vi "Teststand Post Sub Steps Read_FA_FE_FF_Frame STP_Engine.vi"(9 "Socket No":u16=1, 10 "STP Data in":T1={"ECU CAN Port"="CAN1", "CMD"=130, "CAN Write Data"=[], "Frame"="FE_FRAME_LOG", "Log"=TRUE} {"CMD" items=["TSW_VERSION(130)"=130, "WAIT_EVENT(132)"=132, "SEQUENCER(133)"=133, "TSW_RESET(150)"=150, "CONFIG_ECU(151)"=151, "TEST_CORE (152)"=152, "TEST_WATCHDOG (153)"=153, "TEST_MONITORING (154)"=154, "READ_MEMORY (162)"=162, "WRITE_ERASE_MEMORY (164)"=164, "COMM_EXTERNAL (190)"=190, "COMM_INTERNAL (195)"=195, "GET_ANALOG_INPUT (210)"=210, "GET_DIGITAL_INPUT (211)"=211, "GET_FREQUENCY_INPUT (212)"=212, "TEST_INPUT_STRUCTURE (214)"=214, "GENERATE_OUTPUT_SIGNAL (220)"=220, "GENERATE_SYNCHRONIZED_OUTPUT_SIGNALS (221)"=221, "eDCU_Specific (250)"=250]; "CAN Write Data" format="%.0x"}, 11 "Sequence Context In":refnum<k7>) -> (0 "error out":errorcluster, 1 "STP Error":T3, 2 "STP Data Out":T4, 3 "Report Text":string)   [LabVIEW 2023, in "LTT_TeststandSteptypes.lvlib"]
uses:
  LTT_TeststandSteptypes.lvlib
  Control/STP Out Data.ctl
  HardwareAbstractionLayer_LVOOP/CAN/CAN Application Protocols/STP Protocol_class/Ctrls/STP Error Cluster.ctl
  Control/STP Frame Data.ctl
  HardwareAbstractionLayer_LVOOP/CAN/CAN Application Protocols/STP Protocol_class/Ctrls/STP CMD.ctl
  HardwareAbstractionLayer_LVOOP/Report/Report_class/Control/All Log Details.ctl
  HardwareAbstractionLayer_LVOOP/Report/Report_class/Control/UUT Test Info.ctl
  HardwareAbstractionLayer_LVOOP/Report/Report_class/Control/FE FRAME LOG.ctl
  HardwareAbstractionLayer_LVOOP/Report/Report_class/Control/FF FRAME LOG.ctl
  HardwareAbstractionLayer_LVOOP/Report/Report_class/Control/LIMIT TABLE.ctl
  HardwareAbstractionLayer_LVOOP/Report/Report_class/Control/ERROR LOG APPEND.ctl
  HardwareAbstractionLayer_LVOOP/Report/Report_class/Control/ERROR LOG.ctl
  HardwareAbstractionLayer_LVOOP/Report/Report_class/Control/FA FRAME LOG.ctl
  HardwareAbstractionLayer_LVOOP/Report/Report_class/Control/TEST RESULT LOG APPEND.ctl
  HardwareAbstractionLayer_LVOOP/Report/Report_class/Control/TEST RESULT LOG.ctl
  HardwareAbstractionLayer_LVOOP/Report/Report_class/Control/SYSTEM LOG.ctl
  HardwareAbstractionLayer_LVOOP/Report/Report_class/Control/Temperature LOG.ctl
  HardwareAbstractionLayer_LVOOP/Report/Report_class/Control/POWER STATUS.ctl
  HardwareAbstractionLayer_LVOOP/Report/Report_class/Control/CYCLE_DURATION_LOG.ctl
  HardwareAbstractionLayer_LVOOP/CAN/CAN Application Protocols/STP Protocol_class/Ctrls/STP Input Data.ctl
  HardwareAbstractionLayer_LVOOP/CAN/CAN Application Protocols/STP Protocol_class/Ctrls/STP Output Data.ctl
  <vilib>/addons/TestStand/_TSUtility.llb/TestStand - Get Property Value (Number {Unsigned 32-bit Integer}).vi
  <vilib>/addons/TestStand/_TSUtility.llb/TestStand - Get Property Value (Number).vi
  HardwareAbstractionLayer_LVOOP/CAN/CAN Application Protocols/STP Protocol_class/STP Protocol.lvclass
  HardwareAbstractionLayer_LVOOP/Database/Database.lvclass
  HardwareAbstractionLayer_LVOOP/Report/Report_class/Report.lvclass
panel:
  out "RequestTimeout?":bool
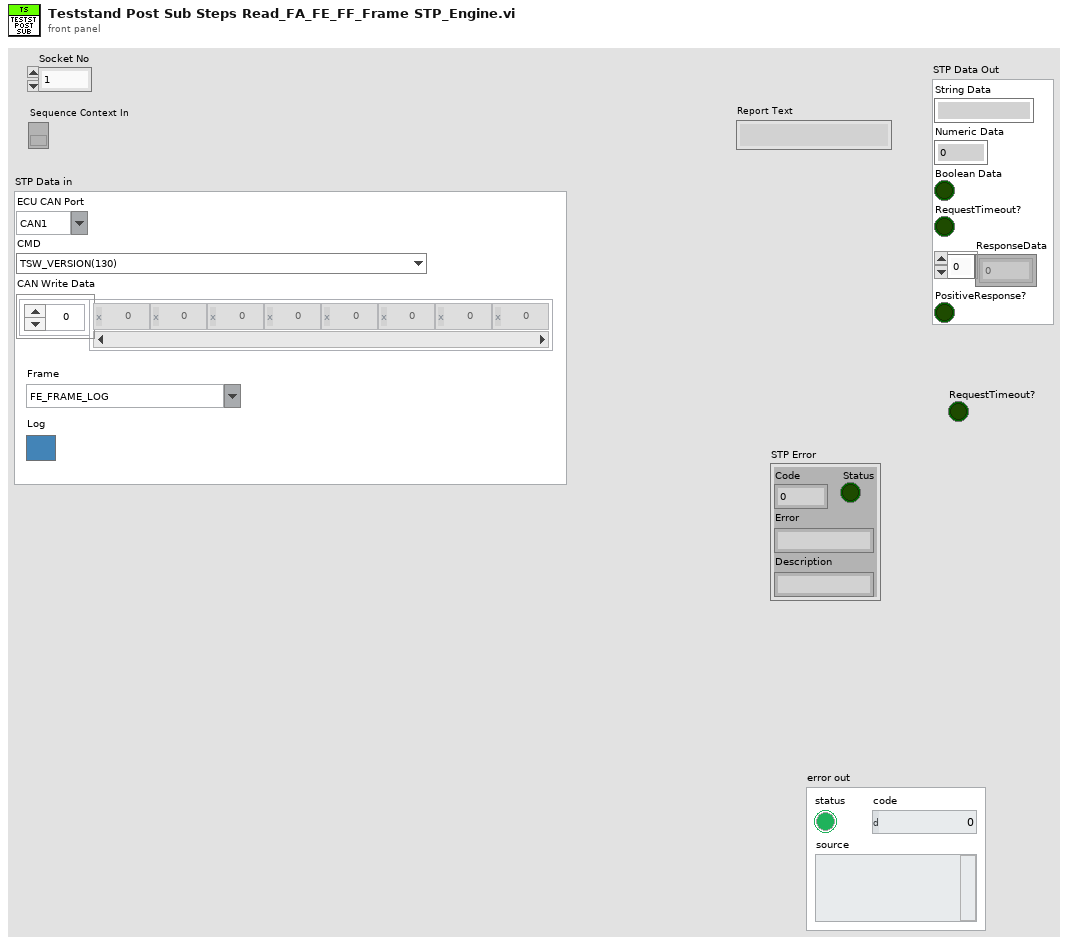
[diagram p1: front panel]
types:
  T1 = typedef "LTT_TeststandSteptypes.lvlib/STP Frame Data.ctl" = cluster{"ECU CAN Port":string, "CMD":T2, "CAN Write Data":u8[], "Frame":string, "Log":bool}
  T2 = typedef "HardwareAbstractionLayer_LVOOP.lvlib/CAN Application Protocols Lib.lvlib/STP Protocol.lvclass/STP CMD.ctl" = u8
  T3 = typedef "HardwareAbstractionLayer_LVOOP.lvlib/CAN Application Protocols Lib.lvlib/STP Protocol.lvclass/STP Error Cluster.ctl" = cluster{"Status":bool, "Code":u8, "Error":string, "Description":string}
  T4 = typedef "LTT_TeststandSteptypes.lvlib/STP Out Data.ctl" = cluster{"String Data":string, "Numeric Data":dbl, "Boolean Data":bool, "RequestTimeout?":bool, "ResponseData":u8[], "PositiveResponse?":bool}
  T5 = typedef "HardwareAbstractionLayer_LVOOP.lvlib/Report.lvclass/All Log Details.ctl" = cluster{"UUT_TEST_INFO":T6, "FE_FRAME_LOG":T7, "FF_FRAME_LOG":T8, "LIMIT_TABLE":T9, "ERROR LOG Append":T10, "FA_FRAME_LOG":T12, "Socket No":u16, "TEST RESULT LOG Append":T13, "SYSTEM_LOG":T15, "Temperature log":T16, "POWER_STATUS":T17, "CYCLE_DURATION_LOG":T18}
  T6 = typedef "HardwareAbstractionLayer_LVOOP.lvlib/Report.lvclass/UUT Test Info.ctl" = cluster{"ID":string, "STATION_ID":string, "TEST_SOCKET_INDEX":string, "UUT_SERIAL_NUMBER":string, "TSW_VER":string, "VAL_SW_VER":string, "PROJECT_NAME":string, "PRODUCT_NAME":string, "PRODUCT_VARIANT":string, "TEST_NAME":string, "TEST_PHASE":string, "TEST_DESCRIPTION":string, "TEMP_CHAMBER_NAME":string, "START_DATE_TIME":string, "STOP_DATE_TIME ":string, "START_CYCLE_COUNT":string, "STOP_CYCLE_COUNT":string, "EXECUTION_TIME":string, "UUT_STATUS":string, "UUT_ERROR_CODE":string, "UUT_ERROR_MESSAGE":string, "TEST_SEQUENCE":string}
  T7 = typedef "HardwareAbstractionLayer_LVOOP.lvlib/Report.lvclass/FE FRAME LOG.ctl" = cluster{"ID":string, "UUT_TEST_INFO":string, "DATE_TIME":string, "CYCLE_NUMBER":string, "TEST_MODE":string, "CHAMBER_TEMP":string, "CAN_FRAME_RX":string, "Test Mode":u32, "LV_PPS_VOLTAGE":string, "LV_PPS_CURRENT":string, "HV_PPS_VOLTAGE":string, "HV_PPS_CURRENT":string, "SOCKET_NUMBER":string, "CAN_FRAME_RX_NO_OFF_BYTE":string}
  T8 = typedef "HardwareAbstractionLayer_LVOOP.lvlib/Report.lvclass/FF FRAME LOG.ctl" = cluster{"ID":string, "UUT_TEST_INFO":string, "DATE_TIME":string, "CYCLE_NUMBER":string, "TEST_MODE":string, "CAN_FRAME_RX":string, "CHAMBER_TEMP":string, "TestMode":u32, "SOCKET_NUMBER":string, "CAN_FRAME_RX_NO_OFF_BYTE":string}
  T9 = typedef "HardwareAbstractionLayer_LVOOP.lvlib/Report.lvclass/LIMIT TABLE.ctl" = cluster{"ID":string, "PRODUCT_NAME":string, "PRODUCT_VARIANT":string, "TEST_MODE":string, "PARAMETER_NAME":string, "COMPARISON_TYPE":string, "LOW_LIMIT":string, "HIGH_LIMIT":string, "UNIT":string, "ERROR_MESSSAGE":string, "SEVERITY":string}
  T10 = typedef "HardwareAbstractionLayer_LVOOP.lvlib/Report.lvclass/ERROR LOG APPEND.ctl" = T11[]
  T11 = typedef "HardwareAbstractionLayer_LVOOP.lvlib/Report.lvclass/ERROR LOG.ctl" = cluster{"ID":string, "UUT_TEST_INFO":string, "DATE_TIME":string, "CYCLE_NUMBER":string, "TEST_MODE":string, "SIGNAL_NAME":string, "SIGNAL_VALUE":string, "UNIT":string, "COMPARISON_VALUE":string, "ERROR_MESSAGE":string, "FRAME_TYPE":string, "LIMITID":string, "SOCKET_NUMBER":string}
  T12 = typedef "HardwareAbstractionLayer_LVOOP.lvlib/Report.lvclass/FA FRAME LOG.ctl" = cluster{"UUT_TEST_INFO":string, "CAN_FRAME_RX":string, "CAN_FRAME_RX_NO_OFF_BYTE":string}
  T13 = typedef "HardwareAbstractionLayer_LVOOP.lvlib/Report.lvclass/TEST RESULT LOG APPEND.ctl" = T14[]
  T14 = typedef "HardwareAbstractionLayer_LVOOP.lvlib/Report.lvclass/TEST RESULT LOG.ctl" = cluster{"ID":string, "UUT_TEST_INFO":string, "DATE_TIME":string, "CYCLE_NUMBER":string, "TEST_MODE":string, "SIGNAL_NAME":string, "SIGNAL_VALUE":string, "COMPARISON_VALUE":string, "ERROR_MESSAGE":string, "FRAME_TYPE":string, "LIMITID":string, "TEST_RESULT":string, "SOCKET_NUMBER":string}
  T15 = typedef "HardwareAbstractionLayer_LVOOP.lvlib/Report.lvclass/SYSTEM LOG.ctl" = cluster{"ID ":string, "DATE_TIME":string, "CYCLE_NUMBER":string, "TEST_MODE":string, "ERROR_MESSAGE":string}
  T16 = typedef "HardwareAbstractionLayer_LVOOP.lvlib/Report.lvclass/Temperature LOG.ctl" = cluster{"TEST_MODE":string, "CYCLE_NUMBER":string, "TEMPERATURE":cluster{"LV_PPS_TEMPERATURE":dbl, "HV_PPS1_TEMPERATURE":dbl, "HV_PPS2_TEMPERATURE":dbl, "HV_PPS3_TEMPERATURE":dbl, "HV_PPS4_TEMPERATURE":dbl, "HV_PPS5_TEMPERATURE":dbl, "HV_PPS6_TEMPERATURE":dbl, "CHAMBER_TEMPERATURE":dbl, "LOAD_U1_TEMPERATURE":dbl, "LOAD_V1_TEMPERATURE":dbl, "LOAD_W1_TEMPERATURE":dbl, "LOAD_U2_TEMPERATURE":dbl, "LOAD_V2_TEMPERATURE":dbl, "LOAD_W2_TEMPERATURE":dbl, "LOAD_U3_TEMPERATURE":dbl, "LOAD_V3_TEMPERATURE":dbl, "LOAD_W3_TEMPERATURE":dbl}, "Temperature Inrange":cluster{"LVPPS_Trip?":bool, "HVPPS1_Trip?":bool, "HVPPS2_Trip?":bool, "HVPPS3_Trip?":bool, "HVPPS4_Trip?":bool, "HVPPS5_Trip?":bool, "HVPPS6_Trip?":bool, "Chamber_Trip?":bool}}
  T17 = typedef "HardwareAbstractionLayer_LVOOP.lvlib/Report.lvclass/POWER STATUS.ctl" = cluster{"TEST_MODE":string, "CYCLE_NUMBER":string, "TYPE_POWER":string, "STATE":string}
  T18 = typedef "HardwareAbstractionLayer_LVOOP.lvlib/Report.lvclass/CYCLE_DURATION_LOG.ctl" = cluster{"CYCLE_NUMBER":string}
  T19 = typedef "HardwareAbstractionLayer_LVOOP.lvlib/CAN Application Protocols Lib.lvlib/STP Protocol.lvclass/STP Input Data.ctl" = cluster{"TxID":u32, "RxID":u32, "CMD":T2, "RQ Data":u8[], "+veResponseCode":u8, "ResponseTimeout (S)":dbl}
  T20 = typedef "HardwareAbstractionLayer_LVOOP.lvlib/CAN Application Protocols Lib.lvlib/STP Protocol.lvclass/STP Output Data.ctl" = cluster{"ResponseData":u8[], "ResponseData(ASCII)":string, "PositiveResponse?":bool, "STP Error":T3}
  T21 = typedef "HardwareAbstractionLayer_LVOOP.lvlib/CAN HAL Lib.lvlib/CAN.lvclass/CAN Init Ctrl.ctl" = cluster{"XNET Interface":refnum<k21>, "Baud Rate":u64, "CAN:Termination":u32, "Echo Transmit?":bool, "scope (normal)":T22}
  T22 = typedef "XNET Control Scope.ctl" = u32
  T23 = cluster{"Refnum out":refnum<k21>, "CAN Init Data":T21, "CAN_RxID":u32, "CAN_TxID":u32, "Timeout":dbl}
  T24 = typedef "HardwareAbstractionLayer_LVOOP.lvlib/Report.lvclass/Result FGV Data.ctl" = cluster{"Project Name":string, "Product Name":string, "Product Varient":string, "Test Name":string, "Test Phase":string, "Test Description":string, "Temp Chamber Name":string, "Schema":string, "Total No of Cycles":u32, "Current Cycle Number":u32, "Cycle Duration":u32, "Current Test Mode":string}
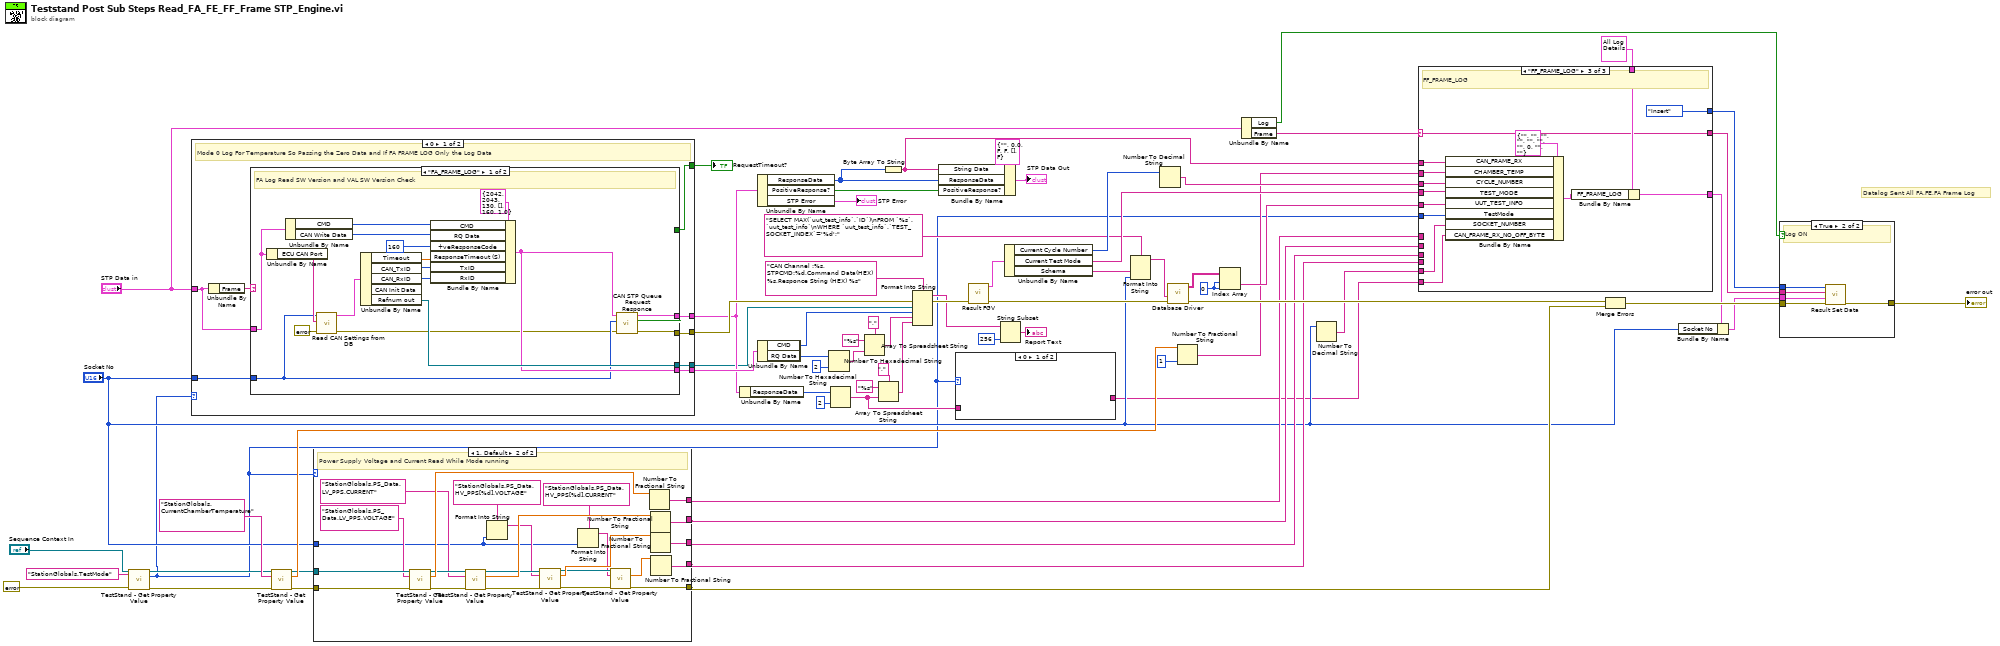
[diagram p0: block diagram]
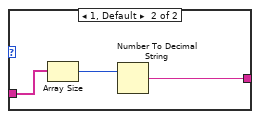
[diagram p3: hidden frame]
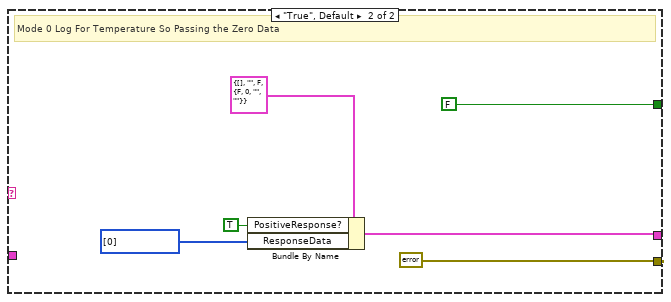
[diagram p5: hidden frame]
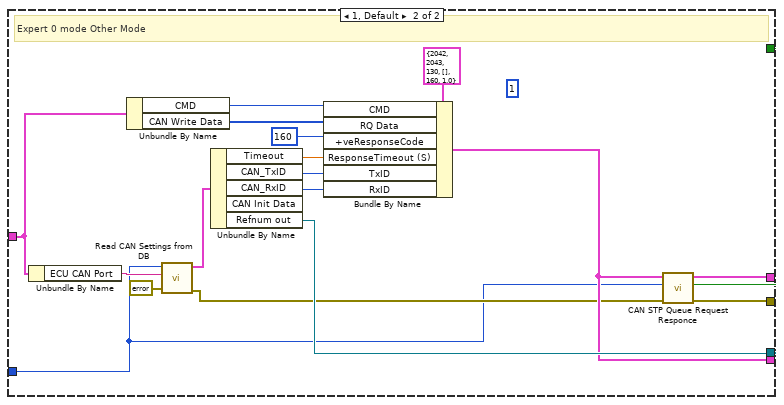
[diagram p6: hidden frame]
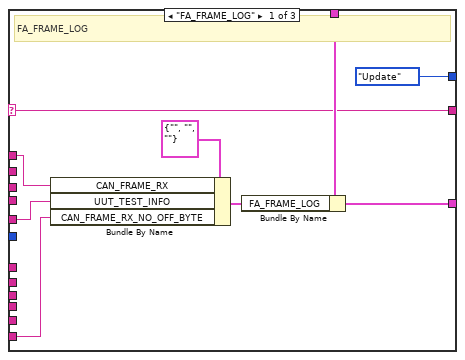
[diagram p7: hidden frame]
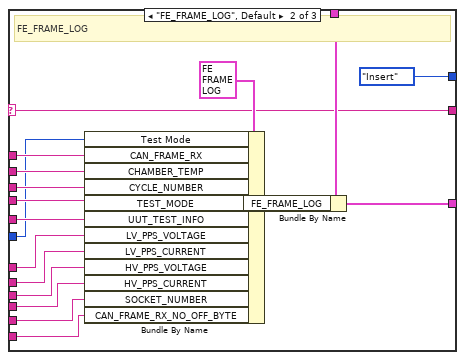
[diagram p8: hidden frame]
diagram:
  w58 = 0 ("disabled index (col)")
  # "Datalog Sent All FA,FE,FA Frame Log"
  n1 = call-poly <vilib>:"TestStand - Get Property Value.vi"("Sequence Context In"="Sequence Context In", "Lookup String"="StationGlobals.TestMode", "error in (no error)"=errorcluster {"status"=FALSE, "code"=0, "source"=""}) -> ("Sequence Context Out"=w20:refnum<k7>, "Value"=w3:u32, "error out"=w21:errorcluster)  [unwired: 10 in]
  n2 = case shown="0" w3 {
    tunnel: "STP Data in" -> [w74 w116]
    tunnel: [w79 w107] -> w41
    tunnel: [w76 w109] -> w38
    tunnel: [w78 w106] -> w37
    tunnel: [w77 w111] -> w31
    tunnel: "Socket No" -> [w75 w105]
    tunnel: [w72 w104] -> w2
    frame 0 {
      # "Mode 0 Log For Temperature So Passing the Zero Data and If FA FRAME LOG Only the Log Data"
      n3 = Unbundle By Name(w74) -> ("Frame"=w73:string)
      n4 = case shown="\"FA_FRAME_LOG\"" w73 {
        tunnel: [w82 errorcluster {"status"=FALSE, "code"=0, "source"=""} ("value out")] -> w79
        tunnel: [w81 w101] -> w78
        tunnel: w74 -> [w87 _]
        tunnel: [w86 _] -> w77
        tunnel: [w85 _] -> w76
        tunnel: w75 -> [w84 _]
        tunnel: [w80 FALSE ("RequestTimeout?")] -> w72
        frame "FA_FRAME_LOG" {
          # "FA Log Read SW Version and VAL SW Version Check"
          n5 = Unbundle By Name(w87) -> ("ECU CAN Port"=w93:string)
          n6 = Unbundle By Name(w87) -> ("CMD"=w96:T2, "CAN Write Data"=w95:u8[])
          n7 = call "Read CAN Settings from DB.vi"("error in"=errorcluster {"status"=FALSE, "code"=0, "source"=""}, "ECU CAN Port"=w93, "Socket No"=w84) -> ("error out"=w83:errorcluster, "Read CAN Setting"=w91:T23)  [unwired: 7 in]
          n8 = Unbundle By Name(w91) -> ("Timeout"=w90:dbl, "CAN_TxID"=w89:u32, "CAN_RxID"=w88:u32, "Refnum out"=w86:refnum<k21>)  [unwired: 1 out]
          n9 = Bundle By Name(cluster=T19 {"TxID"=2042, "RxID"=2043, "CMD"=130, "RQ Data"=[], "+veResponseCode"=160, "ResponseTimeout (S)"=1.0} ("STP Input Data"), "CMD"=w96, "RQ Data"=w95, "+veResponseCode"=u8 160, "ResponseTimeout (S)"=w90, "TxID"=w89, "RxID"=w88) -> (w85:T19)
          n10 = call "CAN STP Queue Request Responce.vi"("error in (no error)"=w83, "Socket No"=w84, "STP Input Data"=w85) -> ("error out"=w82:errorcluster, "RequestTimeout?"=w80:bool, "STP Output Data"=w81:T20)  [unwired: 6 in]
        }
        frame "True", Default {
          # "Mode 0 Log For Temperature So Passing the Zero Data"
          n11 = Bundle By Name(cluster=T20 {"ResponseData"=[], "ResponseData(ASCII)"="", "PositiveResponse?"=FALSE, "STP Error"={"Status"=FALSE, "Code"=0, "Error"="", "Description"=""}} ("STP Output Data"), "PositiveResponse?"=TRUE, "ResponseData"=u8[] [0]) -> (w101:T20)
        }
      }
    }
    frame 1, Default {
      (unwired) 1
      # "Expert 0 mode Other Mode"
      n12 = Unbundle By Name(w116) -> ("ECU CAN Port"=w117:string)
      n13 = Unbundle By Name(w116) -> ("CMD"=w120:T2, "CAN Write Data"=w119:u8[])
      n14 = call "Read CAN Settings from DB.vi"("error in"=errorcluster {"status"=FALSE, "code"=0, "source"=""}, "ECU CAN Port"=w117, "Socket No"=w105) -> ("error out"=w108:errorcluster, "Read CAN Setting"=w114:T23)  [unwired: 7 in]
      n15 = Unbundle By Name(w114) -> ("Timeout"=w110:dbl, "CAN_TxID"=w113:u32, "CAN_RxID"=w112:u32, "Refnum out"=w111:refnum<k21>)  [unwired: 1 out]
      n16 = Bundle By Name(cluster=T19 {"TxID"=2042, "RxID"=2043, "CMD"=130, "RQ Data"=[], "+veResponseCode"=160, "ResponseTimeout (S)"=1.0} ("STP Input Data"), "CMD"=w120, "RQ Data"=w119, "+veResponseCode"=u8 160, "ResponseTimeout (S)"=w110, "TxID"=w113, "RxID"=w112) -> (w109:T19)
      n17 = call "CAN STP Queue Request Responce.vi"("error in (no error)"=w108, "Socket No"=w105, "STP Input Data"=w109) -> ("error out"=w107:errorcluster, "RequestTimeout?"=w104:bool, "STP Output Data"=w106:T20)  [unwired: 6 in]
    }
  }
  "RequestTimeout?" <- w2
  n18 = call-poly <vilib>:"TestStand - Get Property Value.vi"("Sequence Context In"=w20, "Lookup String"="StationGlobals.CurrentChamberTemperature", "error in (no error)"=w21) -> ("Sequence Context Out"=w15:refnum<k7>, "Value"=w34:dbl, "error out"=w16:errorcluster)  [unwired: 10 in]
  n19 = case shown="1, Default" w3 {
    tunnel: w16 -> [w122 w146]
    tunnel: w15 -> [_ w145]
    tunnel: [_ w143] -> w14
    tunnel: [_ w139] -> w13
    tunnel: [_ w138] -> w12
    tunnel: [_ w137] -> w11
    tunnel: [w122 w136] -> w10
    tunnel: "Socket No" -> [_ w123]
    frame 0 {
    }
    frame 1, Default {
      # "Power Supply Voltage and Current Read While Mode running"
      n20 = call-poly <vilib>:"TestStand - Get Property Value.vi"("Sequence Context In"=w145, "Lookup String"="StationGlobals.PS_Data.LV_PPS.VOLTAGE", "error in (no error)"=w146) -> ("Sequence Context Out"=w135:refnum<k7>, "Value"=w144:dbl, "error out"=w134:errorcluster)  [unwired: 10 in]
      n21 = call-poly <vilib>:"TestStand - Get Property Value.vi"("Sequence Context In"=w135, "Lookup String"="StationGlobals.PS_Data.LV_PPS.CURRENT", "error in (no error)"=w134) -> ("Sequence Context Out"=w131:refnum<k7>, "Value"=w142:dbl, "error out"=w133:errorcluster)  [unwired: 10 in]
      n22 = Format Into String(format string="StationGlobals.PS_Data.HV_PPS[%d].VOLTAGE", w123) -> (resulting string=w126:string)  [unwired: 2 in, 1 out]
      n23 = call-poly <vilib>:"TestStand - Get Property Value.vi"("Sequence Context In"=w131, "Lookup String"=w126, "error in (no error)"=w133) -> ("Sequence Context Out"=w130:refnum<k7>, "Value"=w141:dbl, "error out"=w132:errorcluster)  [unwired: 10 in]
      n24 = Format Into String(format string="StationGlobals.PS_Data.HV_PPS[%d].CURRENT", w123) -> (resulting string=w124:string)  [unwired: 2 in, 1 out]
      n25 = call-poly <vilib>:"TestStand - Get Property Value.vi"("Sequence Context In"=w130, "Lookup String"=w124, "error in (no error)"=w132) -> ("Value"=w140:dbl, "error out"=w136:errorcluster)  [unwired: 10 in, 1 out]
      n26 = Number To Fractional String(number=w144) -> (F-format string=w143:string)  [unwired: 3 in]
      n27 = Number To Fractional String(number=w142) -> (F-format string=w139:string)  [unwired: 3 in]
      n28 = Number To Fractional String(number=w141) -> (F-format string=w138:string)  [unwired: 3 in]
      n29 = Number To Fractional String(number=w140) -> (F-format string=w137:string)  [unwired: 3 in]
    }
  }
  n30 = Unbundle By Name(w37) -> ("ResponseData"=w36:u8[])
  n31 = Unbundle By Name(w37) -> ("ResponseData"=w67:u8[], "PositiveResponse?"=w30:bool, "STP Error"=→"STP Error":T3)
  n32 = Unbundle By Name(w38) -> ("CMD"=w52:T2, "RQ Data"=w44:u8[])
  n33 = Number To Hexadecimal String(1:i16 2 ("width (-)"), 2:w44) -> (0:w48:string[])
  n34 = Number To Hexadecimal String(1:i16 2 ("width (-)"), 2:w36) -> (0:w5:string[])
  n35 = Array To Spreadsheet String(delimiter (Tab)=",", array=w48, 3:"%s" ("format string")) -> (spreadsheet string=w50:string)
  n36 = Array To Spreadsheet String(delimiter (Tab)=",", array=w5, 3:"%s" ("format string")) -> (spreadsheet string=w42:string)
  n37 = Byte Array To String(unsigned byte array=w67) -> (string=w68:string)
  n38 = Format Into String(format string="CAN Channel :%s, STPCMD:%d,Command Data(HEX) %s,Responce String (HEX) %s", error in=w41, w31, w52, w50, w42) -> (resulting string=w39:string, error out=w40:errorcluster)  [unwired: 1 in]
  n39 = Bundle By Name(cluster=T4 {"String Data"="", "Numeric Data"=0.0, "Boolean Data"=FALSE, "RequestTimeout?"=FALSE, "ResponseData"=[], "PositiveResponse?"=FALSE} ("STP Data Out"), "String Data"=w68, "ResponseData"=w67, "PositiveResponse?"=w30) -> (→"STP Data Out":T4)
  n40 = case shown="0" w3 {
    tunnel: w5 -> [_ w149]
    tunnel: [_ w147] -> w4
    frame 0 {
    }
    frame 1, Default {
      n41 = Array Size(array=w149) -> (size(s)=w148:i32)
      n42 = Number To Decimal String(number=w148) -> (decimal integer string=w147:string)  [unwired: 1 in]
    }
  }
  n43 = call "Result FGV.vi"("error in"=w40) -> ("error out"=w29:errorcluster, "Result FGV Data Out"=w64:T24)  [unwired: 9 in]
  n44 = String Subset(string=w39, length (rest)=256 ("length (rest)")) -> (substring=→"Report Text":string)  [unwired: 1 in]
  n45 = Unbundle By Name(w64) -> ("Current Cycle Number"=w63:u32, "Current Test Mode"=w62:string, "Schema"=w56:string)
  n46 = Format Into String(format string="SELECT MAX(`uut_test_info`.`ID`)\nFROM `%s`.`uut_test_info`\nWHERE `uut_test_info`.`TEST_SOCKET_INDEX`='%d';", w56, "Socket No") -> (resulting string=w60:string)  [unwired: 2 in, 1 out]
  n47 = Number To Decimal String(number=w63) -> (decimal integer string=w53:string)  [unwired: 1 in]
  n48 = call "Database Driver.vi"("error in"=w29, "SQL query"=w60) -> ("error out"=w57:errorcluster, "data"=w59:string[][])  [unwired: 6 in, 2 out]
  n49 = Number To Fractional String(number=w34, precision (6)=i16 1) -> (F-format string=w27:string)  [unwired: 2 in]
  n50 = Index Array(array=w59, index (row)=w58, index (col)=w58) -> (element=w54:string)
  n51 = Unbundle By Name("STP Data in") -> ("Log"=w1:bool, "Frame"=w55:string)
  n52 = Number To Decimal String(number="Socket No") -> (decimal integer string=w9:string)  [unwired: 1 in]
  n53 = case shown="\"FF_FRAME_LOG\"" w55 {
    selector: w55 -> [w153 w169 w183]
    tunnel: w68 -> [w157 w167 w180]
    tunnel: [w158 w175 w190] -> w19
    tunnel: w53 -> [_ w173 w187]
    tunnel: w62 -> [_ w172 w186]
    tunnel: w54 -> [w152 w166 w179]
    tunnel: w27 -> [_ w171 w185]
    tunnel: T5 {"UUT_TEST_INFO"={"ID"="", "STATION_ID"="", "TEST_SOCKET_INDEX"="", "UUT_SERIAL_NUMBER"="", "TSW_VER"="", "VAL_SW_VER"="", "PROJECT_NAME"="", "PRODUCT_NAME"="", "PRODUCT_VARIANT"="", "TEST_NAME"="", "TEST_PHASE"="", "TEST_DESCRIPTION"="", "TEMP_CHAMBER_NAME"="", "START_DATE_TIME"="", "STOP_DATE_TIME "="", "START_CYCLE_COUNT"="", "STOP_CYCLE_COUNT"="", "EXECUTION_TIME"="", "UUT_STATUS"="", "UUT_ERROR_CODE"="", "UUT_ERROR_MESSAGE"="", "TEST_SEQUENCE"=""}, "FE_FRAME_LOG"={"ID"="", "UUT_TEST_INFO"="", "DATE_TIME"="", "CYCLE_NUMBER"="", "TEST_MODE"="", "CHAMBER_TEMP"="", "CAN_FRAME_RX"="", "Test Mode"=0, "LV_PPS_VOLTAGE"="", "LV_PPS_CURRENT"="", "HV_PPS_VOLTAGE"="", "HV_PPS_CURRENT"="", "SOCKET_NUMBER"="", "CAN_FRAME_RX_NO_OFF_BYTE"=""}, "FF_FRAME_LOG"={"ID"="", "UUT_TEST_INFO"="", "DATE_TIME"="", "CYCLE_NUMBER"="", "TEST_MODE"="", "CAN_FRAME_RX"="", "CHAMBER_TEMP"="", "TestMode"=0, "SOCKET_NUMBER"="", "CAN_FRAME_RX_NO_OFF_BYTE"=""}, "LIMIT_TABLE"={"ID"="", "PRODUCT_NAME"="", "PRODUCT_VARIANT"="", "TEST_MODE"="", "PARAMETER_NAME"="", "COMPARISON_TYPE"="", "LOW_LIMIT"="", "HIGH_LIMIT"="", "UNIT"="", "ERROR_MESSSAGE"="", "SEVERITY"=""}, "ERROR LOG Append"=[], "FA_FRAME_LOG"={"UUT_TEST_INFO"="", "CAN_FRAME_RX"="", "CAN_FRAME_RX_NO_OFF_BYTE"=""}, "Socket No"=1, "TEST RESULT LOG Append"=[], "SYSTEM_LOG"={"ID "="", "DATE_TIME"="", "CYCLE_NUMBER"="", "TEST_MODE"="", "ERROR_MESSAGE"=""}, "Temperature log"={"TEST_MODE"="", "CYCLE_NUMBER"="", "TEMPERATURE"={"LV_PPS_TEMPERATURE"=0.0, "HV_PPS1_TEMPERATURE"=0.0, "HV_PPS2_TEMPERATURE"=0.0, "HV_PPS3_TEMPERATURE"=0.0, "HV_PPS4_TEMPERATURE"=0.0, "HV_PPS5_TEMPERATURE"=0.0, "HV_PPS6_TEMPERATURE"=0.0, "CHAMBER_TEMPERATURE"=0.0, "LOAD_U1_TEMPERATURE"=0.0, "LOAD_V1_TEMPERATURE"=0.0, "LOAD_W1_TEMPERATURE"=0.0, "LOAD_U2_TEMPERATURE"=0.0, "LOAD_V2_TEMPERATURE"=0.0, "LOAD_W2_TEMPERATURE"=0.0, "LOAD_U3_TEMPERATURE"=0.0, "LOAD_V3_TEMPERATURE"=0.0, "LOAD_W3_TEMPERATURE"=0.0}, "Temperature Inrange"={"LVPPS_Trip?"=FALSE, "HVPPS1_Trip?"=FALSE, "HVPPS2_Trip?"=FALSE, "HVPPS3_Trip?"=FALSE, "HVPPS4_Trip?"=FALSE, "HVPPS5_Trip?"=FALSE, "HVPPS6_Trip?"=FALSE, "Chamber_Trip?"=FALSE}}, "POWER_STATUS"={"TEST_MODE"="", "CYCLE_NUMBER"="", "TYPE_POWER"="", "STATE"=""}, "CYCLE_DURATION_LOG"={"CYCLE_NUMBER"=""}} ("Set Data") -> [w156 w170 w184]
    tunnel: [w153 w169 w183] -> w25
    tunnel: [enum16{"Insert", "Update"}."Update" ("Action") enum16{"Insert", "Update"}."Insert" ("Action") enum16{"Insert", "Update"}."Insert" ("Action")] -> w24
    tunnel: w3 -> [_ w161 w181]
    tunnel: w14 -> [_ w165 _]
    tunnel: w13 -> [_ w164 _]
    tunnel: w12 -> [_ w163 _]
    tunnel: w11 -> [_ w162 _]
    tunnel: w9 -> [_ w160 w178]
    tunnel: w4 -> [w150 w159 w177]
    frame "FA_FRAME_LOG" {
      # "FA_FRAME_LOG"
      n54 = Bundle By Name(cluster=T12 {"UUT_TEST_INFO"="", "CAN_FRAME_RX"="", "CAN_FRAME_RX_NO_OFF_BYTE"=""} ("FA_FRAME_LOG"), "CAN_FRAME_RX"=w157, "UUT_TEST_INFO"=w152, "CAN_FRAME_RX_NO_OFF_BYTE"=w150) -> (w154:T12)
      n55 = Bundle By Name(cluster=w156, "FA_FRAME_LOG"=w154) -> (w158:T5)
    }
    frame "FE_FRAME_LOG", Default {
      # "FE_FRAME_LOG"
      n56 = Bundle By Name(cluster=T7 {"ID"="", "UUT_TEST_INFO"="", "DATE_TIME"="", "CYCLE_NUMBER"="", "TEST_MODE"="", "CHAMBER_TEMP"="", "CAN_FRAME_RX"="", "Test Mode"=0, "LV_PPS_VOLTAGE"="", "LV_PPS_CURRENT"="", "HV_PPS_VOLTAGE"="", "HV_PPS_CURRENT"="", "SOCKET_NUMBER"="", "CAN_FRAME_RX_NO_OFF_BYTE"=""} ("FE_FRAME_LOG"), "Test Mode"=w161, "CAN_FRAME_RX"=w167, "CHAMBER_TEMP"=w171, "CYCLE_NUMBER"=w173, "TEST_MODE"=w172, "UUT_TEST_INFO"=w166, "LV_PPS_VOLTAGE"=w165, "LV_PPS_CURRENT"=w164, "HV_PPS_VOLTAGE"=w163, "HV_PPS_CURRENT"=w162, "SOCKET_NUMBER"=w160, "CAN_FRAME_RX_NO_OFF_BYTE"=w159) -> (w176:T7)
      n57 = Bundle By Name(cluster=w170, "FE_FRAME_LOG"=w176) -> (w175:T5)
    }
    frame "FF_FRAME_LOG" {
      # "FF_FRAME_LOG"
      n58 = Bundle By Name(cluster=T8 {"ID"="", "UUT_TEST_INFO"="", "DATE_TIME"="", "CYCLE_NUMBER"="", "TEST_MODE"="", "CAN_FRAME_RX"="", "CHAMBER_TEMP"="", "TestMode"=0, "SOCKET_NUMBER"="", "CAN_FRAME_RX_NO_OFF_BYTE"=""} ("FF_FRAME_LOG"), "CAN_FRAME_RX"=w180, "CHAMBER_TEMP"=w185, "CYCLE_NUMBER"=w187, "TEST_MODE"=w186, "UUT_TEST_INFO"=w179, "TestMode"=w181, "SOCKET_NUMBER"=w178, "CAN_FRAME_RX_NO_OFF_BYTE"=w177) -> (w189:T8)
      n59 = Bundle By Name(cluster=w184, "FF_FRAME_LOG"=w189) -> (w190:T5)
    }
  }
  n60 = Merge Errors(w57, w10) -> (w28:errorcluster)
  n61 = Bundle By Name(cluster=w19, "Socket No"="Socket No") -> (w18:T5)
  n62 = case shown="True" w1 {
    tunnel: [w191 w196] -> w70
    tunnel: w28 -> [w191 w195]
    tunnel: w25 -> [_ w194]
    tunnel: w24 -> [_ w193]
    tunnel: w18 -> [_ w192]
    frame False {
      # "Log Off"
    }
    frame True {
      # "Log ON"
      n63 = call "Result Set Data.vi"("error in"=w195, "Set Data"=w192, "Table Name"=w194, "Action"=w193) -> ("error out"=w196:errorcluster)  [unwired: 7 in]
    }
  }
  "error out" <- w70
